vi "main.vi"() -> ()   [LabVIEW 2017]
uses:
  loop_state.ctl
  <vilib>/Instr/_visa.llb/VISA Open Access Mode.ctl
panel:
  out "error out 3":errorcluster
  out "error out 2":errorcluster
  out "error out":errorcluster
  in  "GotoFlag":bool
  in  "Goto":bool
  in  "Numeric Control":dbl
  in  "OK Button":bool
  in  "Current(A)":dbl min=0.0 max=3.2
  in  "Voltage(V)":dbl min=0.0 max=32.0
  in  "Exit Button":bool
  in  "Threshold Force(N)":dbl
  in  "Down Speed(mm/min)":dbl=0.5 min=0.5 max=1100.0
  in  "Up Speed(mm/min)":dbl=0.5 min=0.5 max=1100.0
  in  "Boolean 3":bool=TRUE
  in  "Up Button":bool
  in  "Down Button":bool
  in  "Zero Force":bool
  in  "Zero Travel":bool
  out "Full Duration":bool
  out "Waveform Chart":T1(graph)
  out "dt":i32
  in  "Sampling Rate":dbl
  in  "Power Supply":refnum<visa-resource-name>
  in  "Mark-10":refnum<visa-resource-name>
  in  "Record File Path":path
  out "Up":bool
  out "Heater Off":bool
  out "Heater On":bool
  out "Down":bool
  in  "Boolean 2":bool=TRUE
  in  "Record Duration":dbl
  in  "Horizontal Pointer Slide":cluster{dbl, dbl, dbl, dbl, dbl}(slide)={0.0, 0.0, 0.0, 8.938547486033519, 45.754189944134076} scale=0.0..15.0 scale format="%#_6f"
  in  "Record Button":bool
  in  "Stop Button":bool
  # "Heater Off"
  # "Down"
  # "Heater On"
  # "Up"
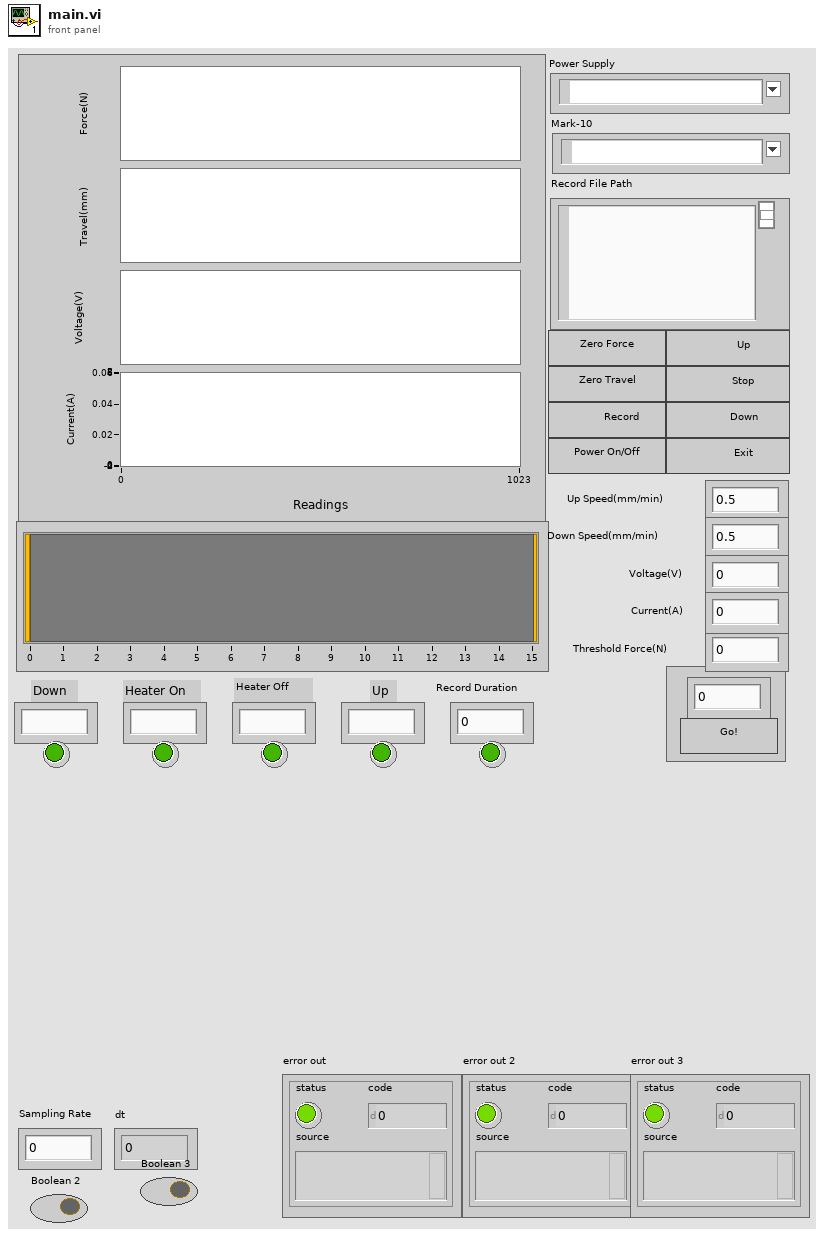
[diagram p1: front panel]
types:
  T1 = cluster{"Numeric":dbl, "Numeric":dbl, "Voltage":dbl, "Current":dbl}
  T2 = typedef "loop_state.ctl" = enum16{"Goto", "On", "Off", "Zero Travel", "Zero Force", "Stop", "Down", "Up", "Acquire", "Log Path Setup", "Initialize"}
  T3 = enum8{"Enabled", "Disabled", "Disabled and Grayed Out"}
  T4 = typedef "VISA Open Access Mode.ctl" = u32
  T5 = cluster{"Array[0]":bool, "Array[1]":bool, "Array[2]":bool, "Array[3]":bool, "Array[4]":bool, bool}
  T6 = cluster{"Array[0]":bool, "Array[1]":bool, "Array[2]":bool, "Array[3]":bool, "Array[4]":bool, "Array[5]":bool, "Array[6]":bool, "Array[7]":bool, "Array[8]":bool}
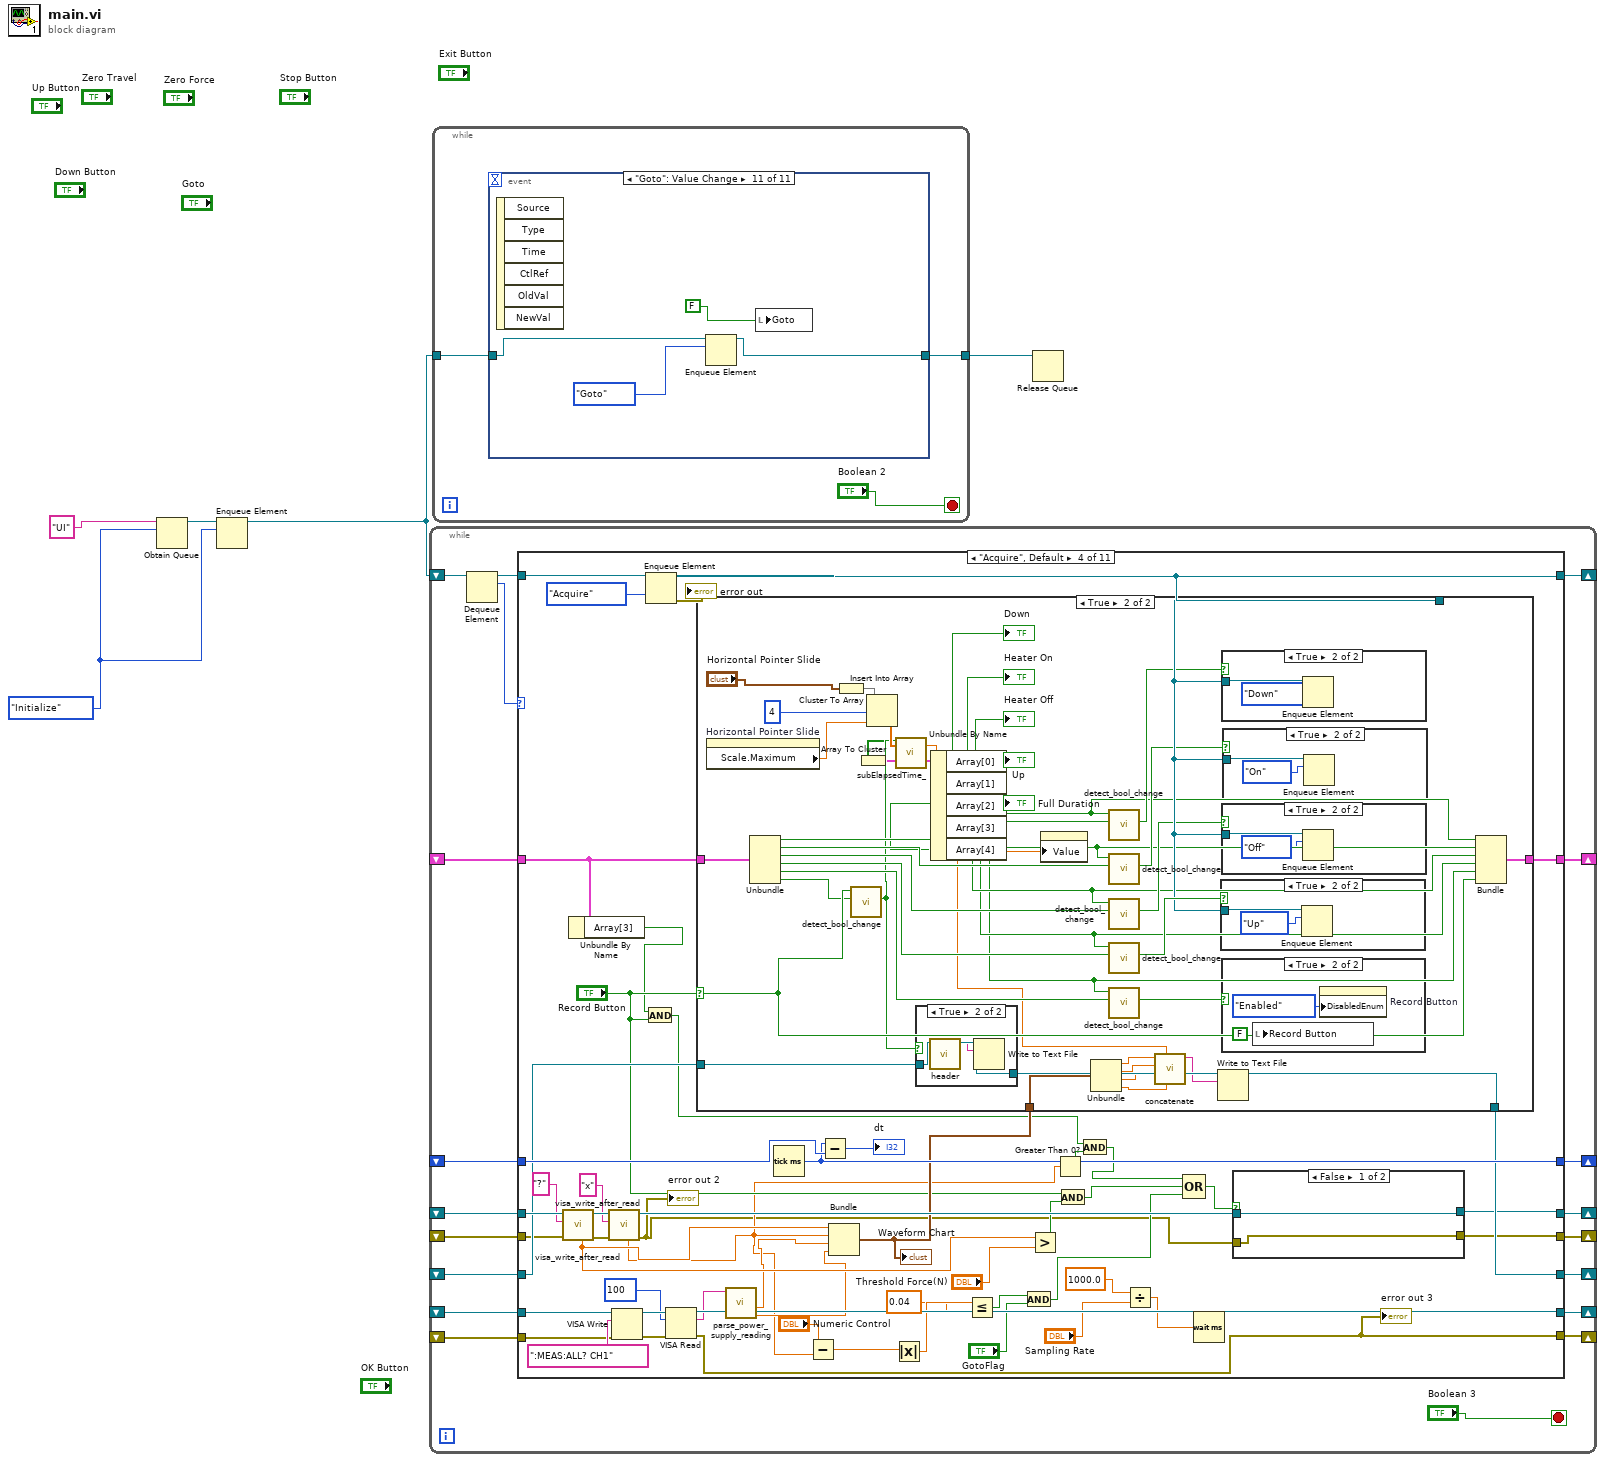
[diagram p0: block diagram]
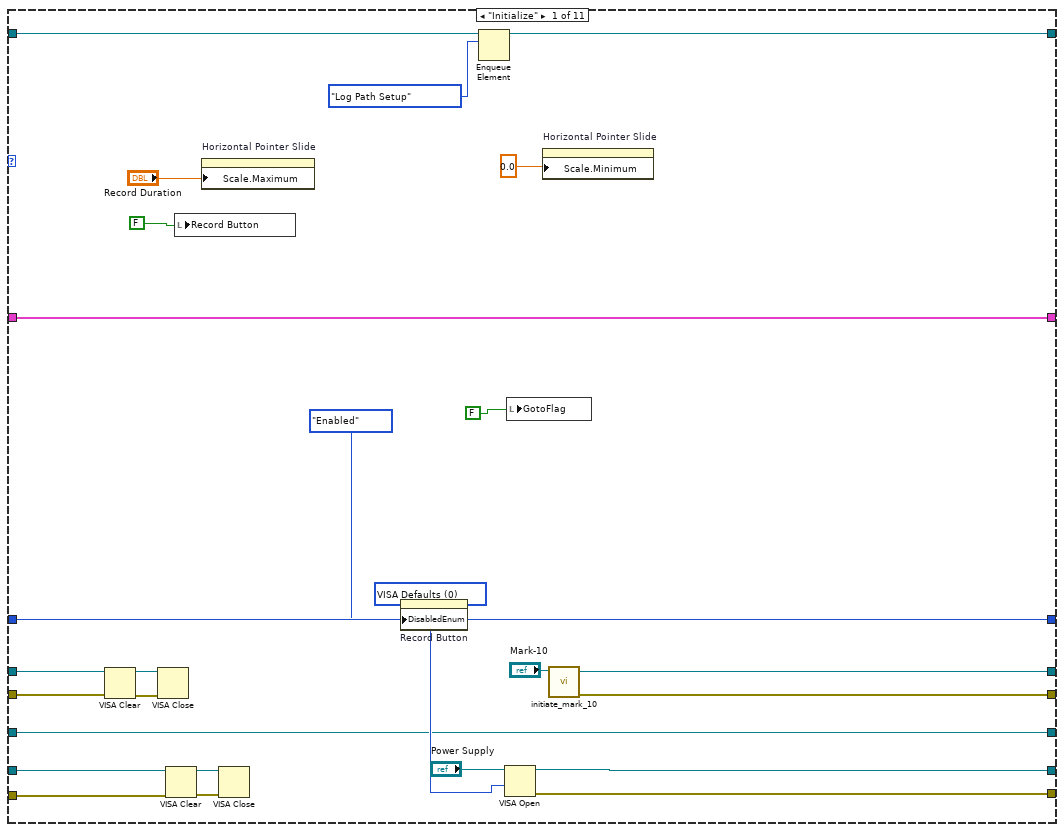
[diagram p2: hidden frame]
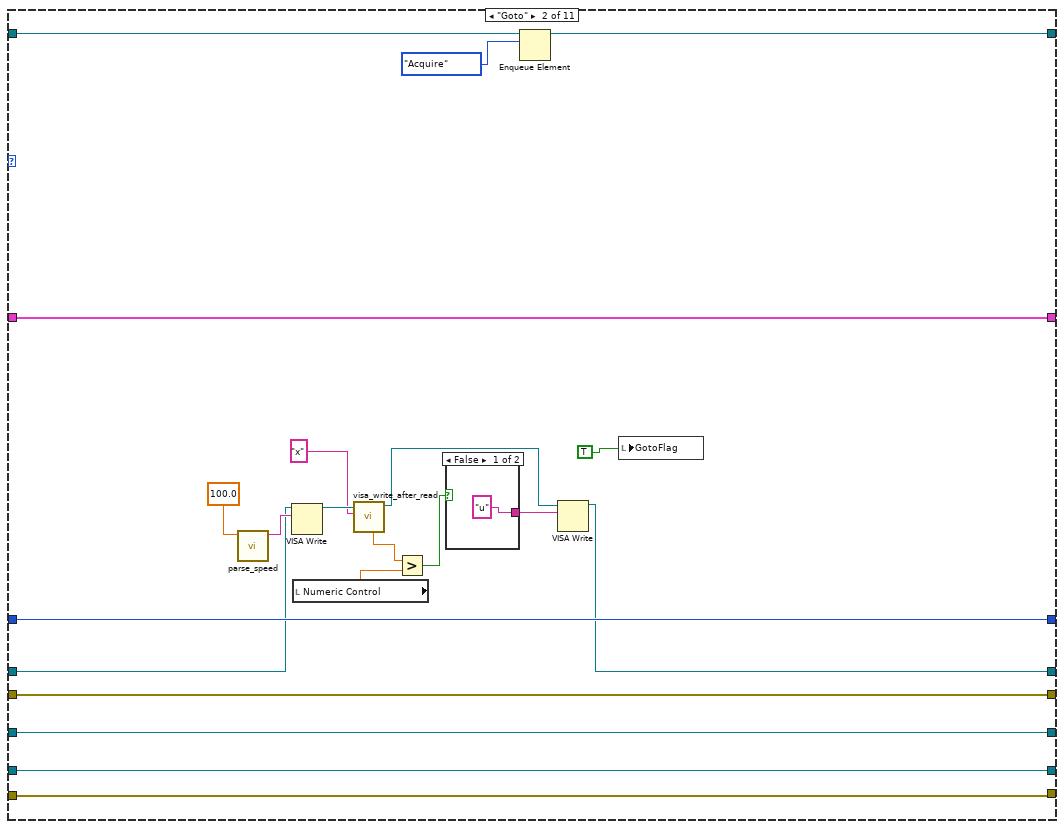
[diagram p3: hidden frame]
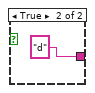
[diagram p4: hidden frame]
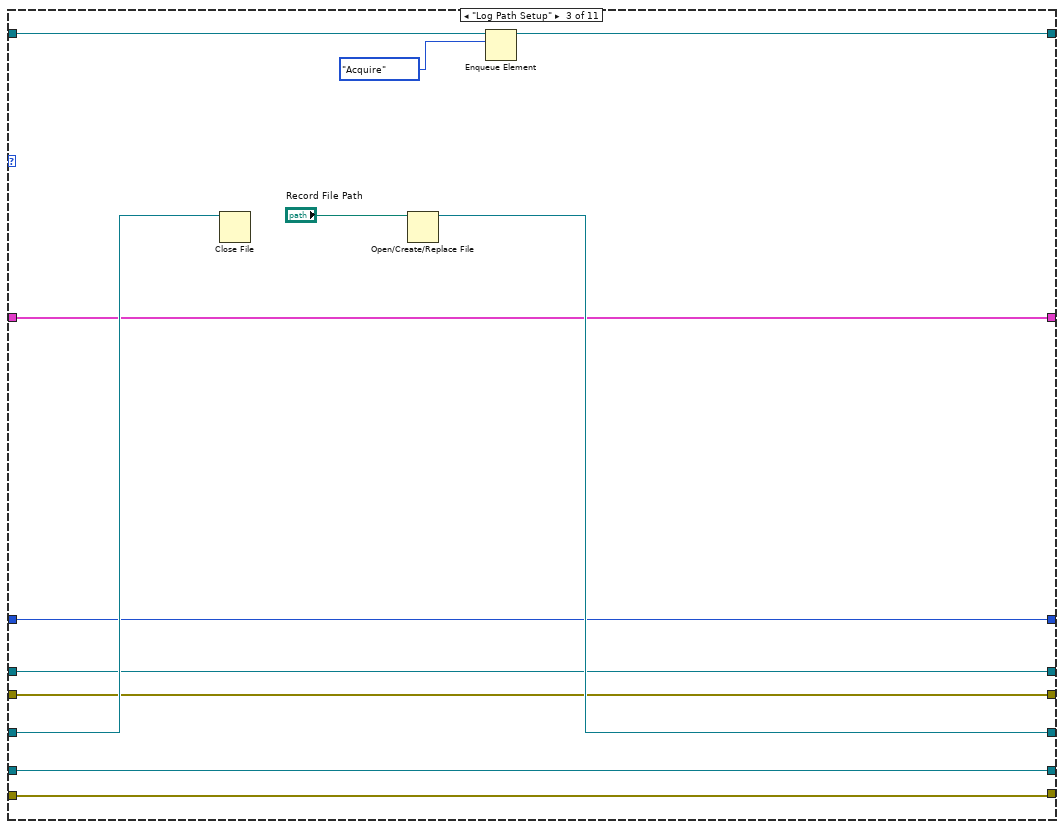
[diagram p5: hidden frame]
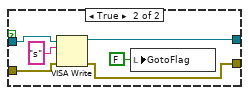
[diagram p6: hidden frame]
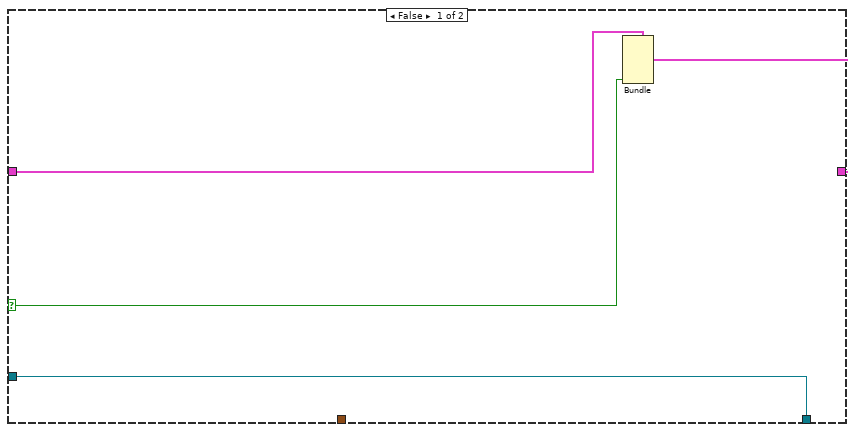
[diagram p7: hidden frame]
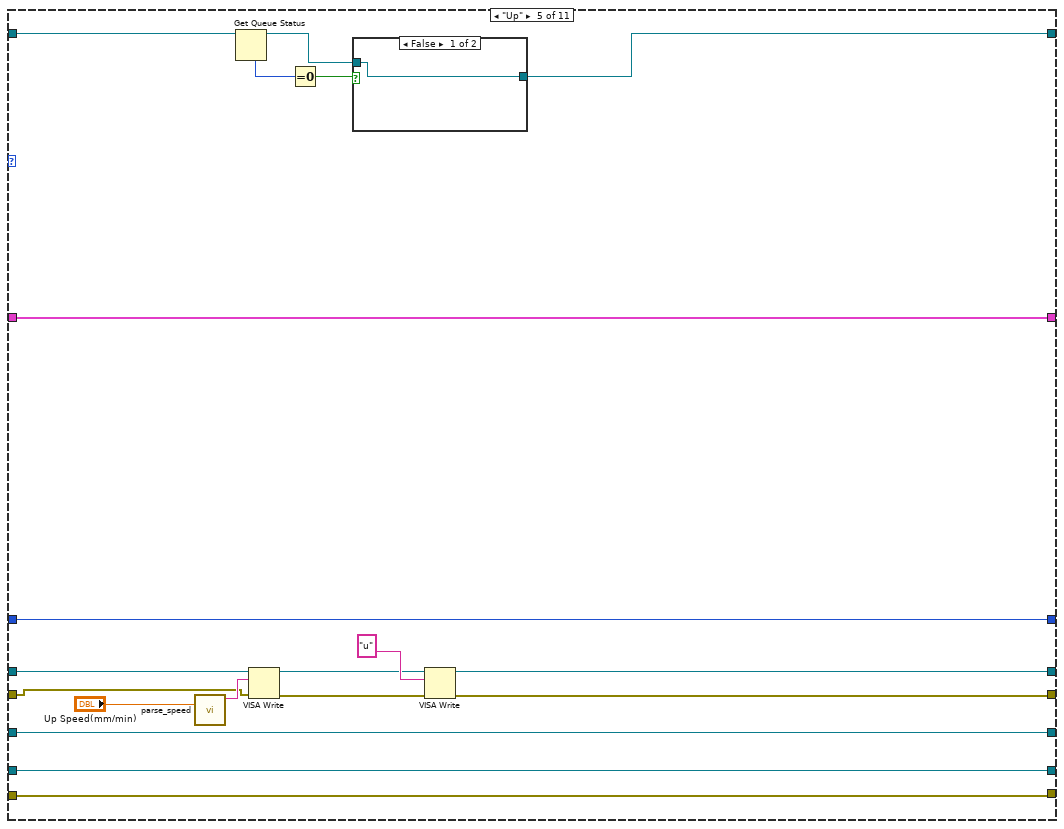
[diagram p14: hidden frame]
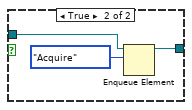
[diagram p15: hidden frame]
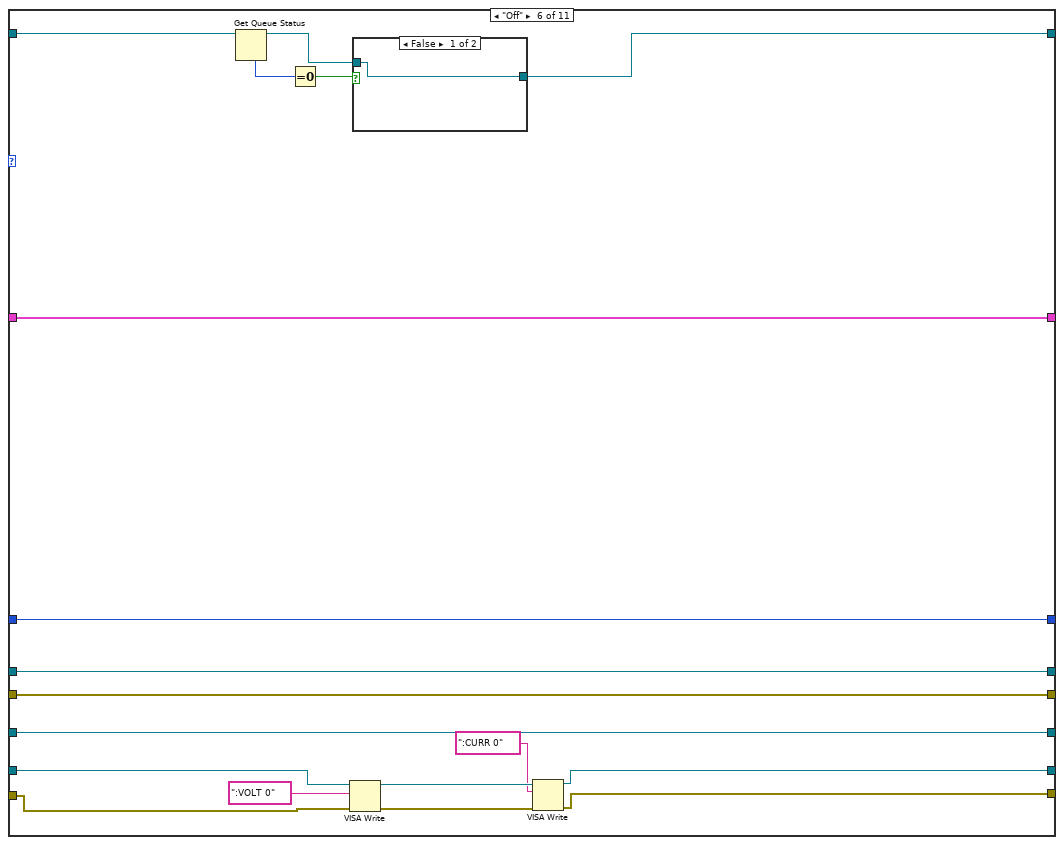
[diagram p16: hidden frame]
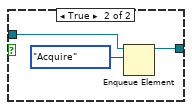
[diagram p17: hidden frame]
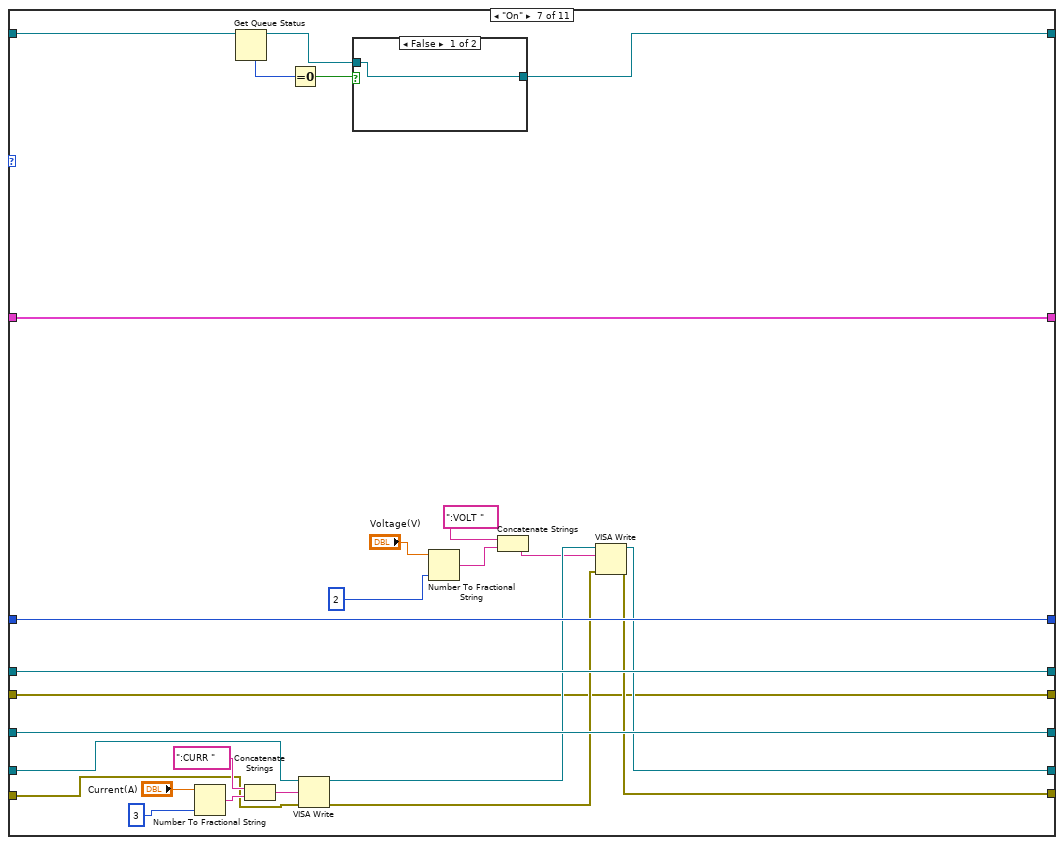
[diagram p18: hidden frame]
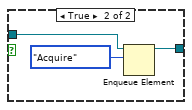
[diagram p19: hidden frame]
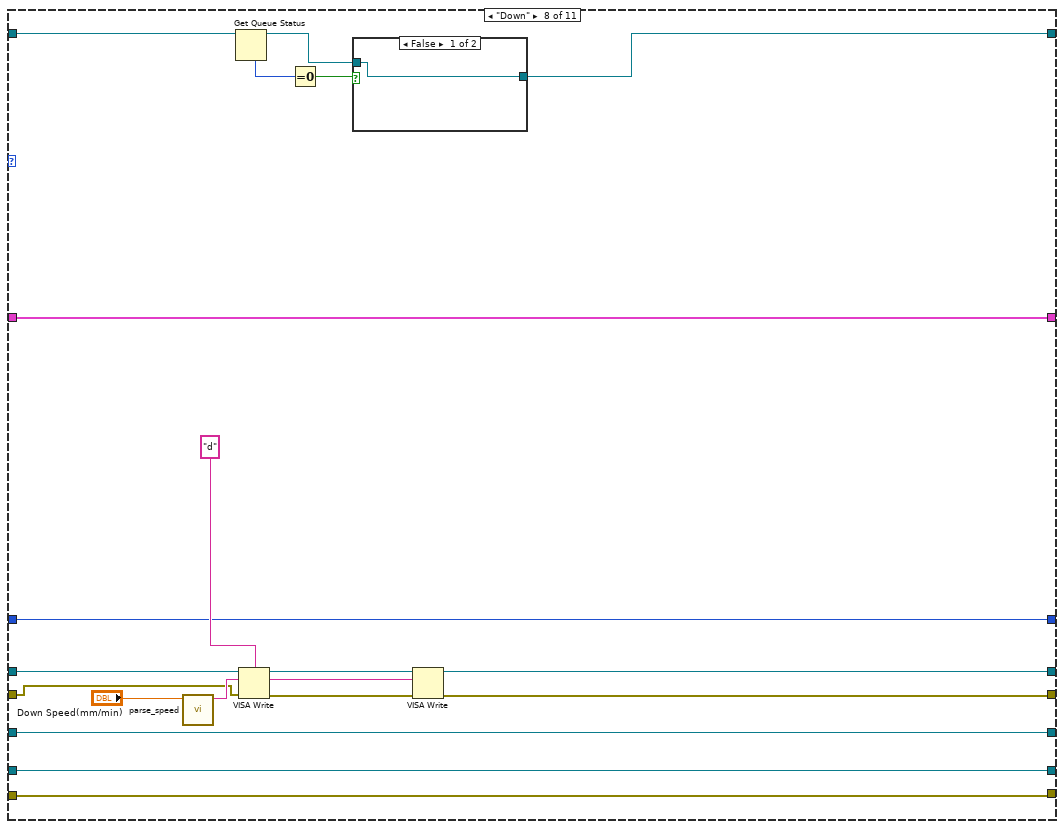
[diagram p20: hidden frame]
diagram:
  w2 = loop_state."Initialize"
  n1 = Obtain Queue(name (unnamed)="UI", element data type=w2) -> (queue out=w3:refnum<queue>)  [unwired: 3 in, 2 out]
  n2 = Enqueue Element(queue=w3, element=w2) -> (queue out=w1:refnum<queue>)  [unwired: 2 in, 2 out]
  n3 = while {
    shift-right: [w24] -> _
    shift-left: _ -> [w22]
    shift-right: [w23] -> _
    shift-left: _ -> [w21]
    shift-right: [w20] -> _
    shift-left: _ -> [w19]
    shift-right: [w18] -> _
    shift-left: _ -> [w17]
    shift-right: [w12] -> _
    shift-left: w1 -> [w14]
    shift-right: [w11] -> _
    shift-left: _ -> [w10]
    shift-right: [w9] -> _
    shift-left: _ -> [w8]
    shift-right: [w7] -> _
    shift-left: _ -> [w6]
    stop <- "Boolean 3" stop-if-true
    n4 = Dequeue Element(queue=w14) -> (queue out=w13:refnum<queue>, element=w15:T2)  [unwired: 2 in, 2 out]
    n5 = case shown="\"Acquire\", Default" w15 {
      tunnel: [w46 w56 w82 w118 w222 w236 w266 w297 w316 w335 w354] -> w24
      tunnel: [w45 w71 w81 w131 w214 w232 w260 w289 w308 w327 w346] -> w23
      tunnel: w22 -> [w42 w57 w82 w139 w210 w236 w266 w286 w306 w325 w344]
      tunnel: w21 -> [w44 w71 w81 w135 w214 w234 w262 w289 w308 w327 w346]
      tunnel: [w40 w70 w84 w121 w215 w239 w269 w290 w309 w328 w347] -> w20
      tunnel: w19 -> [w40 w70 w83 w122 w215 w239 w269 w290 w309 w328 w347]
      tunnel: [w39 w69 w80 w127 w213 w238 w268 w288 w307 w326 w345] -> w18
      tunnel: w17 -> [w39 w69 w80 w128 w213 w238 w268 w288 w307 w326 w345]
      tunnel: w13 -> [w35 w68 w79 w126 w221 w244 w274 w296 w315 w334 w353]
      tunnel: [w34 w67 w78 w123 w217 w240 w270 w292 w311 w330 w349] -> w12
      tunnel: [w32 w65 w76 w125 w208 w237 w267 w283 w305 w324 w343] -> w11
      tunnel: w10 -> [w32 w65 w76 w109 w208 w237 w267 w283 w305 w324 w343]
      tunnel: [w30 w52 w75 w89 w205 w230 w249 w280 w303 w322 w341] -> w9
      tunnel: w8 -> [w29 w52 w75 w92 w207 w230 w249 w282 w304 w323 w342]
      tunnel: [w28 w51 w74 w86 w204 w227 w250 w279 w302 w321 w340] -> w7
      tunnel: w6 -> [w27 w51 w74 w88 w204 w229 w252 w279 w302 w321 w340]
      frame "Initialize" {
        w50 = T4 0 items=["VISA Defaults"=0, "Exclusive Lock"=1, "Load Configured Settings"=4] ("Access Mode")
        n6 = VISA Clear(VISA resource name=w42, error in (no error)=w29) -> (VISA resource name out=w41:refnum<visa-resource-name>, error out=w26:errorcluster)
        n7 = VISA Close(VISA resource name=w41, error in (no error)=w26) -> ()  [unwired: 1 out]
        n8 = VISA Clear(VISA resource name=w44, error in (no error)=w27) -> (VISA resource name out=w43:refnum<visa-resource-name>, error out=w25:errorcluster)
        n9 = local write "Record Button"(FALSE) -> ()
        n10 = property on="Horizontal Pointer Slide" class="Slide (strict)"("Scale.Maximum"="Record Duration") -> ()  [unwired: 2 in, 2 out]
        n11 = VISA Close(VISA resource name=w43, error in (no error)=w25) -> ()  [unwired: 1 out]
        n12 = property on="Record Button" class="Bool (strict)"("DisabledEnum"=T3."Enabled" ("Disabled")) -> ()  [unwired: 2 in, 2 out]
        n13 = Enqueue Element(queue=w35, element=loop_state."Log Path Setup") -> (queue out=w34:refnum<queue>)  [unwired: 2 in, 2 out]
        n14 = VISA Open(access mode=w50, VISA resource name="Power Supply") -> (VISA resource name=w45:refnum<visa-resource-name>, error out=w28:errorcluster)  [unwired: 3 in]
        n15 = local write "GotoFlag"(FALSE) -> ()
        n16 = property on="Horizontal Pointer Slide" class="Slide (strict)"("Scale.Minimum"=0.0) -> ()  [unwired: 2 in, 2 out]
        n17 = call "initiate_mark_10.vi"("VISA Refnum in"="Mark-10") -> ("error out"=w30:errorcluster, "VISA Refnum out"=w46:refnum<visa-resource-name>)  [unwired: 9 in]
      }
      frame "Goto" {
        n18 = call "parse_speed.vi"("Up Speed(mm/min)"=100.0) -> ("String"=w64:string)  [unwired: 10 in]
        n19 = VISA Write(VISA resource name=w57, write buffer=w64) -> (VISA resource name out=w62:refnum<visa-resource-name>)  [unwired: 1 in, 2 out]
        n20 = local read "Numeric Control"() -> (w54:dbl)
        n21 = call "visa_write_after_read.vi"("String"="x", "VISA Refnum in"=w62) -> ("VISA Refnum out"=w59:refnum<visa-resource-name>, "Numeric"=w53:dbl)  [unwired: 6 in, 2 out]
        n22 = Greater?(x=w53, y=w54) -> (0:w55:bool)
        n23 = case shown="False" w55 {
          tunnel: ["u" "d"] -> w60
          frame False {
          }
          frame True {
          }
        }
        n24 = Enqueue Element(queue=w68, element=loop_state."Acquire") -> (queue out=w67:refnum<queue>)  [unwired: 2 in, 2 out]
        n25 = VISA Write(VISA resource name=w59, write buffer=w60) -> (VISA resource name out=w56:refnum<visa-resource-name>)  [unwired: 1 in, 2 out]
        n26 = local write "GotoFlag"(TRUE) -> ()
      }
      frame "Log Path Setup" {
        n27 = Close File(refnum=w83) -> ()  [unwired: 1 in, 2 out]
        n28 = Open/Create/Replace File(file path (use dialog)="Record File Path") -> (refnum out=w84:refnum<file>)  [unwired: 5 in, 2 out]
        n29 = Enqueue Element(queue=w79, element=loop_state."Acquire") -> (queue out=w78:refnum<queue>)  [unwired: 2 in, 2 out]
      }
      frame "Acquire", Default {
        n30 = call "visa_write_after_read.vi"("error in (no error)"=w92, "String"="?", "VISA Refnum in"=w139) -> ("error out"=w91:errorcluster, "VISA Refnum out"=w137:refnum<visa-resource-name>, "Numeric"=w116:dbl)  [unwired: 5 in, 1 out]
        n31 = Unbundle By Name(w109) -> ("Array[3]"=w106:bool)
        n32 = call "visa_write_after_read.vi"("error in (no error)"=w91, "String"="x", "VISA Refnum in"=w137) -> ("error out"=w90:errorcluster, "VISA Refnum out"=w119:refnum<visa-resource-name>, "Numeric"=w98:dbl)  [unwired: 5 in, 1 out]
        "error out 2" <- w90
        n33 = VISA Write(VISA resource name=w135, write buffer=":MEAS:ALL? CH1", error in (no error)=w88) -> (VISA resource name out=w133:refnum<visa-resource-name>, error out=w87:errorcluster)  [unwired: 1 out]
        n34 = And(x=w106, y="Record Button") -> (x .and. y?=w105:bool)
        n35 = Enqueue Element(queue=w126, element=loop_state."Acquire") -> (queue out=w123:refnum<queue>, error out=→"error out":errorcluster)  [unwired: 2 in, 1 out]
        n36 = VISA Read(VISA resource name=w133, byte count=100, error in (no error)=w87) -> (VISA resource name out=w131:refnum<visa-resource-name>, read buffer=w130:string, error out=w86:errorcluster)  [unwired: 1 out]
        "error out 3" <- w86
        n37 = call "parse_power_supply_reading.vi"("read buffer 3"=w130) -> ("Current"=w114:dbl, "Voltage"=w115:dbl)  [unwired: 7 in, 2 out]
        n38 = Tick Count (ms)() -> (millisecond timer value=w127:u32)
        n39 = Subtract(x="Numeric Control", y=w98) -> (x-y=w99:dbl)
        n40 = Subtract(x=w127, y=w128) -> (x-y=→"dt":u32)
        n41 = Bundle("Numeric"=w116, "Numeric"=w98, "Voltage"=w115, "Current"=w114) -> (w113:T1)  [unwired: 1 in]
        "Waveform Chart" <- w113
        n42 = case shown="True" "Record Button" {
          selector: "Record Button" -> [w151 w187]
          tunnel: [w150 w188] -> w125
          tunnel: w109 -> [w149 w189]
          tunnel: w123 -> [_ w178]
          tunnel: w122 -> [w148 w172]
          tunnel: [w148 w174] -> w121
          tunnel: w113 -> [_ w173]
          frame False {
            n43 = Bundle(cluster=w149, w151) -> (w150:T5)  [unwired: 5 in]
          }
          frame True {
            n44 = property on="Horizontal Pointer Slide" class="Slide (strict)"() -> ("Scale.Maximum"=w163:dbl)  [unwired: 2 in, 2 out]
            n45 = Unbundle(w189) -> ("Array[0]"=w185:bool, "Array[1]"=w184:bool, "Array[2]"=w183:bool, "Array[3]"=w182:bool, "Array[4]"=w181:bool, w186:bool)
            n46 = Cluster To Array(cluster="Horizontal Pointer Slide") -> (array=w164:dbl[])
            n47 = call "detect_bool_change.vi"("Boolean in"=w186, "Boolean 3"=w187) -> ("x > y?"=w161:bool)  [unwired: 9 in]
            n48 = Insert Into Array(array=w164, index=4, new element=w163) -> (w162:dbl[])
            n49 = call "subElapsedTime_.vi"("Reset"=w161, "Elapsed Time Target"=w162) -> ("Array"=w157:bool[], "Elapsed Time"=w159:dbl)  [unwired: 16 in]
            n50 = Array To Cluster(array=w157) -> (cluster=w158:T6)
            n51 = case shown="True" w161 {
              tunnel: w172 -> [w190 w193]
              tunnel: [w190 w192] -> w171
              frame False {
              }
              frame True {
                n52 = call "header.vi"() -> ("concatenated string"=w191:string)  [unwired: 11 in]
                n53 = Write to Text File(file (use dialog)=w193, text=w191) -> (refnum out=w192:refnum<file>)  [unwired: 2 in, 2 out]
              }
            }
            n54 = Unbundle By Name(w158) -> ("Array[0]"=w156:bool, "Array[1]"=w155:bool, "Array[2]"=w154:bool, "Array[3]"=w153:bool, "Array[4]"=w152:bool)
            "Down" <- w156
            "Heater On" <- w155
            "Heater Off" <- w154
            "Up" <- w153
            "Full Duration" <- w152
            n55 = property class="DigNum (strict)"("Value"=w159) -> ()  [unwired: 2 in, 2 out]
            n56 = Unbundle(w173) -> ("Numeric"=w170:dbl, "Numeric"=w169:dbl, "Voltage"=w168:dbl, "Current"=w167:dbl)
            n57 = call "detect_bool_change.vi"("Boolean in"=w185, "Boolean 3"=w156) -> ("x > y?"=w177:bool)  [unwired: 9 in]
            n58 = call "detect_bool_change.vi"("Boolean in"=w184, "Boolean 3"=w155) -> ("x > y?"=w176:bool)  [unwired: 9 in]
            n59 = call "detect_bool_change.vi"("Boolean in"=w183, "Boolean 3"=w154) -> ("x > y?"=w175:bool)  [unwired: 9 in]
            n60 = call "detect_bool_change.vi"("Boolean in"=w182, "Boolean 3"=w153) -> ("x > y?"=w179:bool)  [unwired: 9 in]
            n61 = call "detect_bool_change.vi"("Boolean in"=w181, "Boolean 3"=w152) -> ("x > y?"=w180:bool)  [unwired: 9 in]
            n62 = call "concatenate.vi"("Numeric Control 2"=w167, "Numeric Control"=w159, "Numeric Control 3"=w168, "Numeric Control 4"=w169, "Numeric Control 5"=w170) -> ("String"=w166:string)  [unwired: 6 in]
            n63 = Write to Text File(file (use dialog)=w171, text=w166) -> (refnum out=w174:refnum<file>)  [unwired: 2 in, 2 out]
            n64 = case shown="True" w179 {
              tunnel: w178 -> [_ w200]
              frame False {
              }
              frame True {
                n65 = Enqueue Element(queue=w200, element=loop_state."Up") -> ()  [unwired: 2 in, 3 out]
              }
            }
            n66 = case shown="True" w177 {
              tunnel: w178 -> [_ w194]
              frame False {
              }
              frame True {
                n67 = Enqueue Element(queue=w194, element=loop_state."Down") -> ()  [unwired: 2 in, 3 out]
              }
            }
            n68 = case shown="True" w175 {
              tunnel: w178 -> [_ w198]
              frame False {
              }
              frame True {
                n69 = Enqueue Element(queue=w198, element=loop_state."Off") -> ()  [unwired: 2 in, 3 out]
              }
            }
            n70 = case shown="True" w180 {
              frame False {
              }
              frame True {
                n71 = local write "Record Button"(FALSE) -> ()
                n72 = property on="Record Button" class="Bool (strict)"("DisabledEnum"=T3."Enabled" ("Disabled")) -> ()  [unwired: 2 in, 2 out]
              }
            }
            n73 = case shown="True" w176 {
              tunnel: w178 -> [_ w196]
              frame False {
              }
              frame True {
                n74 = Enqueue Element(queue=w196, element=loop_state."On") -> ()  [unwired: 2 in, 3 out]
              }
            }
            n75 = Bundle("Array[0]"=w156, "Array[1]"=w155, "Array[2]"=w154, "Array[3]"=w153, "Array[4]"=w152, w187) -> (w188:T5)  [unwired: 1 in]
          }
        }
        n76 = Absolute Value(x=w99) -> (abs(x)=w95:dbl)
        n77 = Less Or Equal?(x=w95, y=0.04) -> (x <= y?=w104:bool)
        n78 = And(x=w104, y="GotoFlag") -> (x .and. y?=w96:bool)
        n79 = Greater?(x=w116, y="Threshold Force(N)") -> (0:w117:bool)
        n80 = Greater Than 0?(x=w98) -> (x > 0?=w108:bool)
        n81 = And(x="Record Button", y=w117) -> (x .and. y?=w101:bool)
        n82 = And(x=w105, y=w108) -> (x .and. y?=w102:bool)
        n83 = Divide(x=1000.0, y="Sampling Rate") -> (x/y=w110:dbl)
        n84 = Compound Arithmetic op=OR(w102, w101, w96) -> (w100:bool)
        n85 = Wait (ms)(milliseconds to wait=w110) -> ()  [unwired: 1 out]
        n86 = case shown="False" w100 {
          tunnel: w119 -> [w141 w146]
          tunnel: [w141 w145] -> w118
          tunnel: w90 -> [w140 w143]
          tunnel: [w140 w142] -> w89
          frame False {
          }
          frame True {
            n87 = VISA Write(VISA resource name=w146, write buffer="s", error in (no error)=w143) -> (VISA resource name out=w145:refnum<visa-resource-name>, error out=w142:errorcluster)  [unwired: 1 out]
            n88 = local write "GotoFlag"(FALSE) -> ()
          }
        }
      }
      frame "Up" {
        n89 = call "parse_speed.vi"("Up Speed(mm/min)"="Up Speed(mm/min)") -> ("String"=w209:string)  [unwired: 10 in]
        n90 = Get Queue Status(queue=w221) -> (queue out=w218:refnum<queue>, # elements in queue=w220:i32)  [unwired: 2 in, 6 out]
        n91 = VISA Write(VISA resource name=w210, write buffer=w209, error in (no error)=w207) -> (VISA resource name out=w211:refnum<visa-resource-name>, error out=w206:errorcluster)  [unwired: 1 out]
        n92 = Equal To 0?(x=w220) -> (x = 0?=w219:bool)
        n93 = case shown="False" w219 {
          tunnel: w218 -> [w223 w225]
          tunnel: [w223 w224] -> w217
          frame False {
          }
          frame True {
            n94 = Enqueue Element(queue=w225, element=loop_state."Acquire") -> (queue out=w224:refnum<queue>)  [unwired: 2 in, 2 out]
          }
        }
        n95 = VISA Write(VISA resource name=w211, write buffer="u", error in (no error)=w206) -> (VISA resource name out=w222:refnum<visa-resource-name>, error out=w205:errorcluster)  [unwired: 1 out]
      }
      frame "Off" {
        n96 = Get Queue Status(queue=w244) -> (queue out=w241:refnum<queue>, # elements in queue=w243:i32)  [unwired: 2 in, 6 out]
        n97 = Equal To 0?(x=w243) -> (x = 0?=w242:bool)
        n98 = VISA Write(VISA resource name=w234, write buffer=":VOLT 0", error in (no error)=w229) -> (VISA resource name out=w233:refnum<visa-resource-name>, error out=w228:errorcluster)  [unwired: 1 out]
        n99 = case shown="False" w242 {
          tunnel: w241 -> [w245 w247]
          tunnel: [w245 w246] -> w240
          frame False {
          }
          frame True {
            n100 = Enqueue Element(queue=w247, element=loop_state."Acquire") -> (queue out=w246:refnum<queue>)  [unwired: 2 in, 2 out]
          }
        }
        n101 = VISA Write(VISA resource name=w233, write buffer=":CURR 0", error in (no error)=w228) -> (VISA resource name out=w232:refnum<visa-resource-name>, error out=w227:errorcluster)  [unwired: 1 out]
      }
      frame "On" {
        n102 = Number To Fractional String(number="Current(A)", precision (6)=3) -> (F-format string=w255:string)  [unwired: 2 in]
        n103 = Get Queue Status(queue=w274) -> (queue out=w271:refnum<queue>, # elements in queue=w273:i32)  [unwired: 2 in, 6 out]
        n104 = Concatenate Strings(":CURR ", w255) -> (w254:string)
        n105 = Equal To 0?(x=w273) -> (x = 0?=w272:bool)
        n106 = VISA Write(VISA resource name=w262, write buffer=w254, error in (no error)=w252) -> (VISA resource name out=w261:refnum<visa-resource-name>, error out=w251:errorcluster)  [unwired: 1 out]
        n107 = case shown="False" w272 {
          tunnel: w271 -> [w275 w277]
          tunnel: [w275 w276] -> w270
          frame False {
          }
          frame True {
            n108 = Enqueue Element(queue=w277, element=loop_state."Acquire") -> (queue out=w276:refnum<queue>)  [unwired: 2 in, 2 out]
          }
        }
        n109 = Number To Fractional String(number="Voltage(V)", precision (6)=2) -> (F-format string=w263:string)  [unwired: 2 in]
        n110 = Concatenate Strings(":VOLT ", w263) -> (w259:string)
        n111 = VISA Write(VISA resource name=w261, write buffer=w259, error in (no error)=w251) -> (VISA resource name out=w260:refnum<visa-resource-name>, error out=w250:errorcluster)  [unwired: 1 out]
      }
      frame "Down" {
        n112 = call "parse_speed.vi"("Up Speed(mm/min)"="Down Speed(mm/min)") -> ("String"=w285:string)  [unwired: 10 in]
        n113 = Get Queue Status(queue=w296) -> (queue out=w293:refnum<queue>, # elements in queue=w295:i32)  [unwired: 2 in, 6 out]
        n114 = VISA Write(VISA resource name=w286, write buffer=w285, error in (no error)=w282) -> (VISA resource name out=w287:refnum<visa-resource-name>, error out=w281:errorcluster)  [unwired: 1 out]
        n115 = Equal To 0?(x=w295) -> (x = 0?=w294:bool)
        n116 = case shown="False" w294 {
          tunnel: w293 -> [w298 w300]
          tunnel: [w298 w299] -> w292
          frame False {
          }
          frame True {
            n117 = Enqueue Element(queue=w300, element=loop_state."Acquire") -> (queue out=w299:refnum<queue>)  [unwired: 2 in, 2 out]
          }
        }
        n118 = VISA Write(VISA resource name=w287, write buffer="d", error in (no error)=w281) -> (VISA resource name out=w297:refnum<visa-resource-name>, error out=w280:errorcluster)  [unwired: 1 out]
      }
      frame "Zero Force" {
        n119 = Get Queue Status(queue=w315) -> (queue out=w312:refnum<queue>, # elements in queue=w314:i32)  [unwired: 2 in, 6 out]
        n120 = Equal To 0?(x=w314) -> (x = 0?=w313:bool)
        n121 = case shown="True" w313 {
          tunnel: w312 -> [w317 w319]
          tunnel: [w317 w318] -> w311
          frame False {
          }
          frame True {
            n122 = Enqueue Element(queue=w319, element=loop_state."Acquire") -> (queue out=w318:refnum<queue>)  [unwired: 2 in, 2 out]
          }
        }
        n123 = VISA Write(VISA resource name=w306, write buffer="R", error in (no error)=w304) -> (VISA resource name out=w316:refnum<visa-resource-name>, error out=w303:errorcluster)  [unwired: 1 out]
      }
      frame "Zero Travel" {
        n124 = Get Queue Status(queue=w334) -> (queue out=w331:refnum<queue>, # elements in queue=w333:i32)  [unwired: 2 in, 6 out]
        n125 = Equal To 0?(x=w333) -> (x = 0?=w332:bool)
        n126 = case shown="False" w332 {
          tunnel: w331 -> [w336 w338]
          tunnel: [w336 w337] -> w330
          frame False {
          }
          frame True {
            n127 = Enqueue Element(queue=w338, element=loop_state."Acquire") -> (queue out=w337:refnum<queue>)  [unwired: 2 in, 2 out]
          }
        }
        n128 = VISA Write(VISA resource name=w325, write buffer="z", error in (no error)=w323) -> (VISA resource name out=w335:refnum<visa-resource-name>, error out=w322:errorcluster)  [unwired: 1 out]
      }
      frame "Stop" {
        n129 = Get Queue Status(queue=w353) -> (queue out=w350:refnum<queue>, # elements in queue=w352:i32)  [unwired: 2 in, 6 out]
        n130 = Equal To 0?(x=w352) -> (x = 0?=w351:bool)
        n131 = case shown="False" w351 {
          tunnel: w350 -> [w355 w357]
          tunnel: [w355 w356] -> w349
          frame False {
          }
          frame True {
            n132 = Enqueue Element(queue=w357, element=loop_state."Acquire") -> (queue out=w356:refnum<queue>)  [unwired: 2 in, 2 out]
          }
        }
        n133 = VISA Write(VISA resource name=w344, write buffer="s", error in (no error)=w342) -> (VISA resource name out=w354:refnum<visa-resource-name>, error out=w341:errorcluster)  [unwired: 1 out]
      }
    }
  }
  n134 = while {
    tunnel: w1 -> [w360]
    tunnel: [w359] -> w5
    stop <- "Boolean 2" stop-if-true
    n135 = event shown="[10] \"Goto\": Value Change" {
      selector: _ -> [_ _ _ _ _ _ _ _ _ _ _]
      dyn-events: _ -> [_ _ _ _ _ _ _ _ _ _ _]
      timeout: _ -> [_ _ _ _ _ _ _ _ _ _ _]
      tunnel: w360 -> [w362 w364 w367 w371 w375 w379 w383 w386 w389 w392 w399]
      tunnel: [w362 w364 w366 w370 w374 w378 w382 w386 w388 w391 w397] -> w359
      event Timeout {
        n136 = event-data() -> ()  [unwired: 1 in, 2 out]
      }
      event "Record Duration": Value Change {
        n137 = event-data() -> ()  [unwired: 1 in, 1 out]
        n138 = local read "Record Duration"() -> (w363:dbl)
        n139 = property on="Horizontal Pointer Slide" class="Slide (strict)"("Scale.Maximum"=w363) -> ()  [unwired: 2 in, 2 out]
      }
      event "Up Button": Value Change {
        n140 = event-data() -> ()  [unwired: 1 in, 1 out]
        n141 = Enqueue Element(queue=w367, element=loop_state."Up") -> (queue out=w366:refnum<queue>)  [unwired: 2 in, 2 out]
        n142 = local write "Up Button"(FALSE) -> ()
      }
      event "Down Button": Value Change {
        n143 = event-data() -> ()  [unwired: 1 in, 1 out]
        n144 = Enqueue Element(queue=w371, element=loop_state."Down") -> (queue out=w370:refnum<queue>)  [unwired: 2 in, 2 out]
        n145 = local write "Down Button"(FALSE) -> ()
      }
      event "Zero Force": Value Change {
        n146 = event-data() -> ()  [unwired: 1 in, 1 out]
        n147 = Enqueue Element(queue=w375, element=loop_state."Zero Force") -> (queue out=w374:refnum<queue>)  [unwired: 2 in, 2 out]
        n148 = local write "Zero Force"(FALSE) -> ()
      }
      event "Zero Travel": Value Change {
        n149 = event-data() -> ()  [unwired: 1 in, 1 out]
        n150 = Enqueue Element(queue=w379, element=loop_state."Zero Travel") -> (queue out=w378:refnum<queue>)  [unwired: 2 in, 2 out]
        n151 = local write "Zero Travel"(FALSE) -> ()
      }
      event "Stop Button": Value Change {
        n152 = event-data() -> ()  [unwired: 1 in, 1 out]
        n153 = Enqueue Element(queue=w383, element=loop_state."Stop") -> (queue out=w382:refnum<queue>)  [unwired: 2 in, 2 out]
        n154 = local write "Stop Button"(FALSE) -> ()
      }
      event "Record Button": Value Change {
        n155 = event-data() -> ()  [unwired: 1 in, 1 out]
        n156 = property on="Record Button" class="Bool (strict)"("DisabledEnum"=T3."Disabled and Grayed Out" ("Disabled")) -> ()  [unwired: 2 in, 2 out]
      }
      event "Record File Path": Value Change {
        n157 = event-data() -> ()  [unwired: 1 in, 1 out]
        n158 = Enqueue Element(queue=w389, element=loop_state."Log Path Setup") -> (queue out=w388:refnum<queue>)  [unwired: 2 in, 2 out]
      }
      event "OK Button": Value Change {
        n159 = event-data() -> ("NewVal"=w393:bool)  [unwired: 1 in, 5 out]
        n160 = case shown="False" w393 {
          tunnel: [loop_state."Off" loop_state."On"] -> w390
          frame False {
          }
          frame True {
          }
        }
        n161 = Enqueue Element(queue=w392, element=w390) -> (queue out=w391:refnum<queue>)  [unwired: 2 in, 2 out]
      }
      event "Goto": Value Change {
        n162 = event-data() -> ()  [unwired: 1 in, 6 out]
        n163 = Enqueue Element(queue=w399, element=loop_state."Goto") -> (queue out=w397:refnum<queue>)  [unwired: 2 in, 2 out]
        n164 = local write "Goto"(FALSE) -> ()
      }
    }
  }
  n165 = Release Queue(queue=w5) -> ()  [unwired: 2 in, 3 out]
